vi "enqueue connection status request.vi"(8 "error in":errorcluster, 10 "app type":T4, 11 "active connection in":T1) -> (0 "error out":errorcluster, 3 "active connection out":T1)   [LabVIEW 2012]
uses:
  typedefs/app type.ctl
  connection manager/typedefs/connection type.ctl
  connection manager/typedefs/tcp connection info.ctl
  connection manager/typedefs/interthread get connection status message.ctl
  typedefs/interthread message.ctl
  typedefs/state queue fglbl actions.ctl
  typedefs/HMI PC thread IDs.ctl
  typedefs/station cDAQ thread IDs.ctl
  typedefs/station AuditHMI thread IDs.ctl
  connection manager/typedefs/active connection.ctl
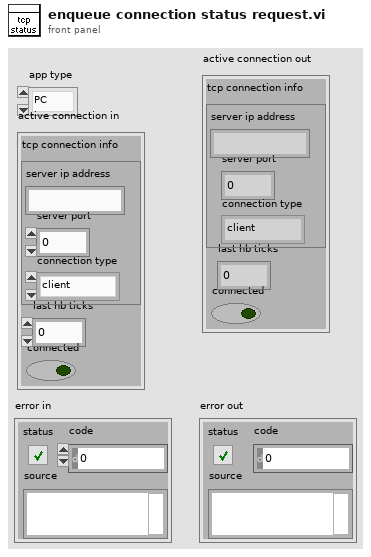
[diagram p1: front panel]
types:
  T1 = typedef "active connection.ctl" = cluster{"tcp connection info":T2, "last hb ticks":u32, "connected":bool}
  T2 = typedef "tcp connection info.ctl" = cluster{"server ip address":string, "server port":i32, "connection type":T3}
  T3 = typedef "connection type.ctl" = enum16{"client", "server"}
  T4 = typedef "app type.ctl" = enum16{"PC", "cDAQ", "AuditHMI"}
  T5 = typedef "HMI PC thread IDs.ctl" = enum16{"hmi main", "file output", "tcp comms", "NVH process"}
  T6 = typedef "station AuditHMI thread IDs.ctl" = enum16{"AuditHMI main", "tcp comms"}
  T7 = typedef "station cDAQ thread IDs.ctl" = enum16{"cDAQ main", "analog input", "eol test exe", "nvh test exe", "tcp comms"}
  T8 = typedef "state queue fglbl actions.ctl" = enum16{"init queues", "get queue ref", "destroy queues"}
  T9 = typedef "interthread message.ctl" = cluster{"destination state":string, "data":variant}
  T10 = typedef "interthread get connection status message.ctl" = cluster{"tcp connection info":T2, "reply-to state":string, "reply-to thread":string, "reply-to app":T4}
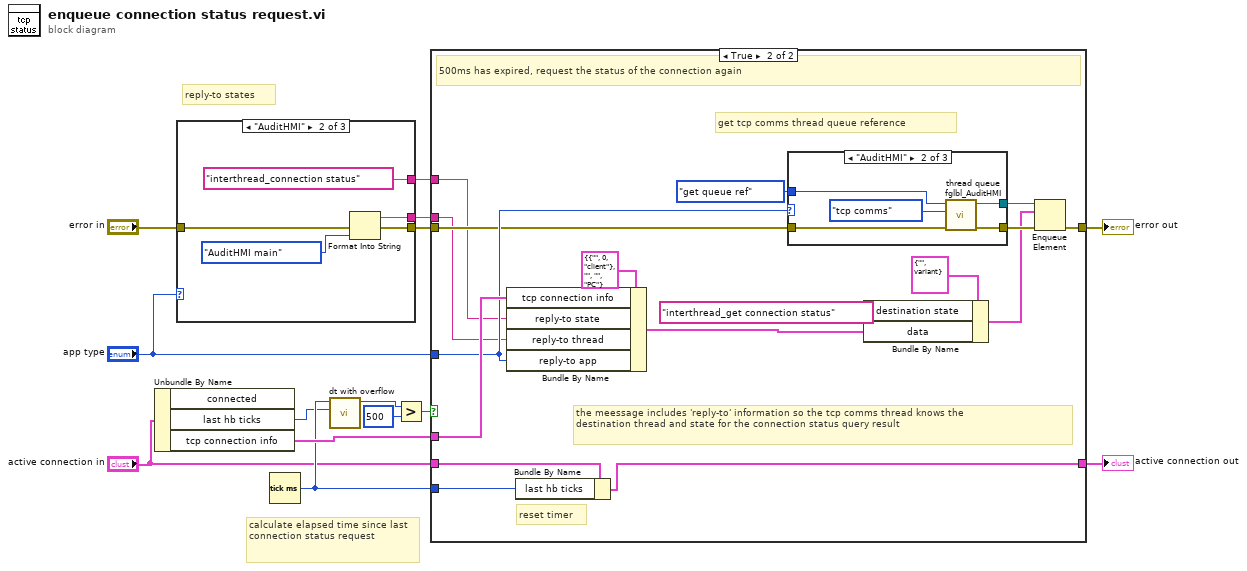
[diagram p0: block diagram]
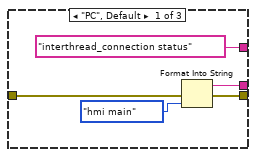
[diagram p2: hidden frame]
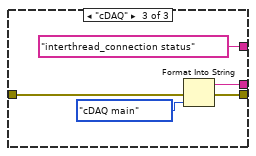
[diagram p3: hidden frame]
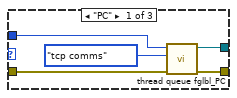
[diagram p5: hidden frame]
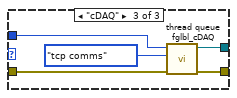
[diagram p6: hidden frame]
diagram:
  # "calculate elapsed time since last connection status request"
  # "reply-to states"
  n1 = Unbundle By Name("active connection in") -> ("last hb ticks"=w2:u32, "tcp connection info"=w10:T2)  [unwired: 1 out]
  n2 = case shown="\"AuditHMI\"" "app type" {
    tunnel: "error in" -> [w19 w24 w28]
    tunnel: [w17 w22 w27] -> w13
    tunnel: [w18 w23 w26] -> w14
    tunnel: ["interthread_connection status" "interthread_connection status" "interthread_connection status"] -> w1
    frame "PC", Default {
      n3 = Format Into String(error in=w19, HMI_PC_thread_IDs."hmi main" ("Station cDAQ Thread Queue")) -> (resulting string=w18:string, error out=w17:errorcluster)  [unwired: 2 in]
    }
    frame "AuditHMI" {
      n4 = Format Into String(error in=w24, station_AuditHMI_thread_IDs."AuditHMI main" ("Station AuditHMI Thread ID")) -> (resulting string=w23:string, error out=w22:errorcluster)  [unwired: 2 in]
    }
    frame "cDAQ" {
      n5 = Format Into String(error in=w28, station_cDAQ_thread_IDs."cDAQ main" ("Station cDAQ Thread Queue")) -> (resulting string=w26:string, error out=w27:errorcluster)  [unwired: 2 in]
    }
  }
  n6 = Tick Count (ms)() -> (millisecond timer value=w9:u32)
  n7 = call "dt with overflow.vi"("t0"=w2, "t1"=w9) -> ("t1-t0"=w3:u32)  [unwired: 9 in]
  n8 = Greater?(x=w3, y=u32 500) -> (0:w5:bool)
  n9 = case shown="True" w5 {
    tunnel: [w31 w46] -> w6
    tunnel: w13 -> [w31 w35]
    tunnel: [w30 w45] -> w7
    tunnel: "active connection in" -> [w30 w38]
    tunnel: w9 -> [_ w44]
    tunnel: w10 -> [_ w43]
    tunnel: "app type" -> [_ w36]
    tunnel: w14 -> [_ w34]
    tunnel: w1 -> [_ w32]
    frame False {
      # "do nothing"
    }
    frame True {
      # "the meessage includes 'reply-to' information so the tcp comms thread knows the\ndestination thread and state for the connection status query result"
      # "reset timer"
      # "get tcp comms thread queue reference"
      # "500ms has expired, request the status of the connection again"
      n10 = Bundle By Name(cluster=T10 {"tcp connection info"={"server ip address"="", "server port"=0, "connection type"=enum."client"}, "reply-to state"="", "reply-to thread"="", "reply-to app"=enum."PC"}, "tcp connection info"=w43, "reply-to state"=w32, "reply-to thread"=w34, "reply-to app"=w36) -> (w39:T10)
      n11 = Bundle By Name(cluster=w38, "last hb ticks"=w44) -> (w45:T1)
      n12 = case shown="\"AuditHMI\"" w36 {
        tunnel: [w50 w56 w63] -> w48
        tunnel: [w51 w57 w61] -> w47
        tunnel: w35 -> [w52 w58 w60]
        tunnel: state_queue_fglbl_actions."get queue ref" ("action") -> [w49 w55 w59]
        frame "PC" {
          n13 = call "thread queue fglbl_PC.vi"("error in (no error)"=w52, "Station cDAQ Thread Queue"=HMI_PC_thread_IDs."tcp comms", "action"=w49) -> ("error out"=w51:errorcluster, "queue out"=w50:refnum<queue>)  [unwired: 6 in, 1 out]
        }
        frame "AuditHMI" {
          n14 = call "thread queue fglbl_AuditHMI.vi"("error in (no error)"=w58, "Station AuditHMI Thread ID"=station_AuditHMI_thread_IDs."tcp comms", "action"=w55) -> ("error out"=w57:errorcluster, "queue out"=w56:refnum<queue>)  [unwired: 6 in, 1 out]
        }
        frame "cDAQ" {
          n15 = call "thread queue fglbl_cDAQ.vi"("error in (no error)"=w60, "Station cDAQ Thread Queue"=station_cDAQ_thread_IDs."tcp comms", "action"=w59) -> ("error out"=w61:errorcluster, "queue out"=w63:refnum<queue>)  [unwired: 6 in, 1 out]
        }
      }
      n16 = Bundle By Name(cluster=T9 {"destination state"="", "data"=variant} ("message"), "destination state"="interthread_get connection status", "data"=w39) -> (w40:T9)
      n17 = Enqueue Element(queue=w48, element=w40, error in (no error)=w47) -> (error out=w46:errorcluster)  [unwired: 1 in, 2 out]
    }
  }
  "active connection out" <- w7
  "error out" <- w6
